vi "is AH bridge.vi"(8 "error in (no error)":errorcluster, 11 "VISA Resource Name":refnum<visa-resource-name>) -> (0 "error out":errorcluster, 2 "is AH?":bool, 3 "VISA Resource Name Out":refnum<visa-resource-name>)   [LabVIEW 2015]
uses:
  GPIB/VISA  Send Receive.vi
panel:
  out "data string out":string
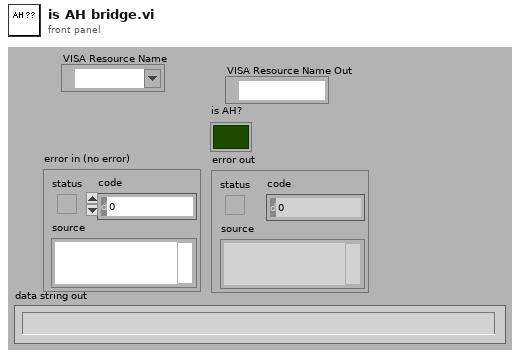
[diagram p1: front panel]
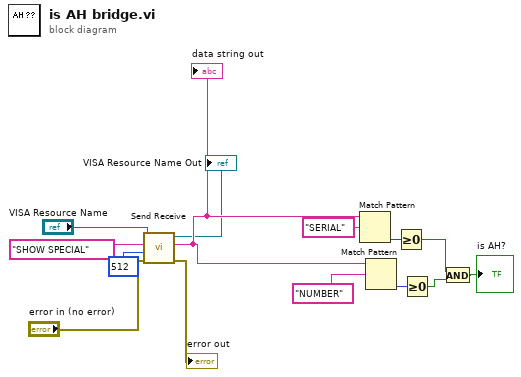
[diagram p0: block diagram]
diagram:
  n1 = call-poly "Send Receive.vi"("error in (no error)"="error in (no error)", "Receive count"=512 ("read count"), "data string in"="SHOW SPECIAL" ("write buffer"), "VISA Resource Name"="VISA Resource Name") -> ("error out"=→"error out":errorcluster, "data string out"=w7:string, "VISA Resource Name Out"=→"VISA Resource Name Out":refnum<visa-resource-name>)  [unwired: 5 in]
  "data string out" <- w7
  n2 = Match Pattern(string=w7, regular expression="SERIAL") -> (offset past match=w11:i32)  [unwired: 4 out]
  n3 = Match Pattern(string=w7, regular expression="NUMBER") -> (offset past match=w8:i32)  [unwired: 4 out]
  n4 = Greater Or Equal To 0?(x=w11) -> (x >= 0?=w10:bool)
  n5 = Greater Or Equal To 0?(x=w8) -> (x >= 0?=w5:bool)
  n6 = And(x=w10, y=w5) -> (x .and. y?=→"is AH?":bool)
